vi "set group info.vi"(8 "error in (no error)":errorcluster, 9 "group info":T1, 10 "id":string, 11 "DSFConfiguration in":refnum<class "DSFConfiguration.lvclass">) -> (0 "error out":errorcluster, 3 "DSFConfiguration out":refnum<class "DSFConfiguration.lvclass">)   [LabVIEW 2017, in "DSFConfiguration.lvclass"]
uses:
  DSFConfiguration.lvclass
  Controls/dsf timing.ctl
  Controls/dsf group.ctl
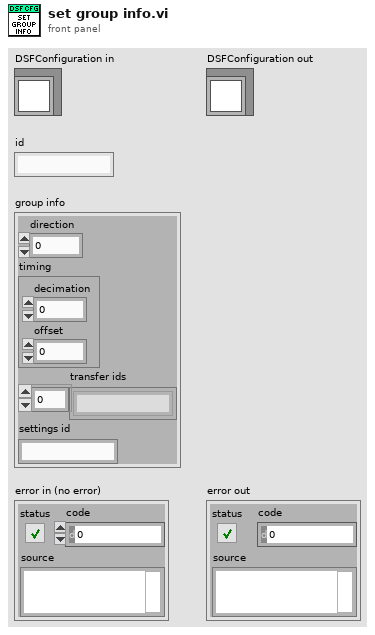
[diagram p1: front panel]
types:
  T1 = typedef "dsf group.ctl" = cluster{"direction":i32, "timing":T2, "transfer ids":string[], "settings id":string}
  T2 = typedef "dsf timing.ctl" = cluster{"decimation":i32, "offset":i32}
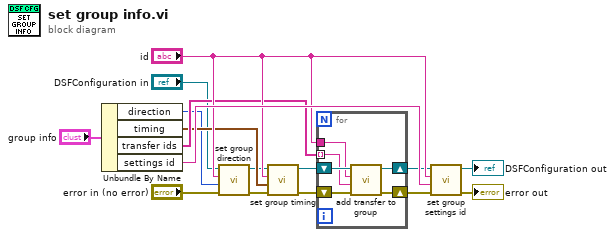
[diagram p0: block diagram]
diagram:
  n1 = Unbundle By Name("group info") -> ("direction"=w5:i32, "timing"=w8:T2, "transfer ids"=w11:string[], "settings id"=w16:string)
  n2 = call "set group direction.vi"("error in (no error)"="error in (no error)", "direction"=w5, "id"="id", "DSFConfiguration in"="DSFConfiguration in") -> ("error out"=w3:errorcluster, "DSFConfiguration out"=w7:refnum<class "DSFConfiguration.lvclass">)  [unwired: 6 in]
  n3 = call "set group timing.vi"("error in (no error)"=w3, "timing"=w8, "id"="id", "DSFConfiguration in"=w7) -> ("error out"=w6:errorcluster, "DSFConfiguration out"=w10:refnum<class "DSFConfiguration.lvclass">)  [unwired: 6 in]
  n4 = for {
    tunnel: "id" -> [w18]
    tunnel: w11 -> [w17] mode=indexing
    shift-right: [w21] -> w9
    shift-left: w6 -> [w22]
    shift-right: [w19] -> w13
    shift-left: w10 -> [w20]
    n5 = call "add transfer to group.vi"("error in (no error)"=w22, "transfer id"=w17, "id"=w18, "DSFConfiguration in"=w20) -> ("error out"=w21:errorcluster, "DSFConfiguration out"=w19:refnum<class "DSFConfiguration.lvclass">)  [unwired: 6 in]
  }
  n6 = call "set group settings id.vi"("error in (no error)"=w9, "settings id"=w16, "id"="id", "DSFConfiguration in"=w13) -> ("error out"=→"error out":errorcluster, "DSFConfiguration out"=→"DSFConfiguration out":refnum<class "DSFConfiguration.lvclass">)  [unwired: 6 in]
